vi "XY Plot Commands W2D.vi"(0 "wavenames":string[](array[string])=["'IV0_summ.itx.0003'[0][0]", "'IV0_summ.itx.0003'[0][1]", "'IV0_summ.itx.0003'[0][2]", "'IV0_summ.itx.0003'[0][3]", "'IV0_summ.itx.0003'[0][4]", "'IV0_summ.itx.0003'[0][5]", "'IV0_summ.itx.0003'[0][6]", "'IV0_summ.itx.0003'[0][7]", "'IV0_summ.itx.0003'[0][8]", "'IV0_summ.itx.0003'[0][9]", "'IV0_summ.itx.0003'[0][10]", "'IV0_summ.itx.0003'[0][11]", "'IV0_summ.itx.0003'[0][12]", "'IV0_summ.itx.0003'[0][13]", "'IV0_summ.itx.0003'[0][14]", "'IV0_summ.itx.0003'[0][15]", "'IV0_summ.itx.0003'[0][16]", "'IV0_summ.itx.0003'[0][17]", "'IV0_summ.itx.0003'[0][18]", "'IV0_summ.itx.0003'[0][19]", "'IV0_summ.itx.0003'[0][20]"], 1 "X label":string="energy (eV)", 2 "Y label":string="amplitude (arb)", 3 "input string":string="Display #wave# vs '#waveX#'\nAppendToGraph #wave# vs '#waveX#'\nLabel bottom \"#labelX#\"\nLabel left \"#labelY#\"\nModifyGraph rgb(#wave#)=(#r#,#g#,#b#)\nLegend/C/N=text0\nModifyGraph mirror=1", 4 "X wave":string="x_") -> (5 "result string":string="Display 'IV0_summ.itx.0003'[0][0] vs 'x_'\nAppendToGraph 'IV0_summ.itx.0003'[0][1] vs 'x_'\nAppendToGraph 'IV0_summ.itx.0003'[0][2] vs 'x_'\nAppendToGraph 'IV0_summ.itx.0003'[0][3] vs 'x_'\nAppendToGraph 'IV0_summ.itx.0003'[0][4] vs 'x_'\nAppendToGraph 'IV0_summ.itx.0003'[0][5] vs 'x_'\nAppendToGraph 'IV0_summ.itx.0003'[0][6] vs 'x_'\nAppendToGraph 'IV0_summ.itx.0003'[0][7] vs 'x_'\nAppendToGraph 'IV0_summ.itx.0003'[0][8] vs 'x_'\nAppendToGraph 'IV0_summ.itx.0003'[0][9] vs 'x_'\nAppendToGraph 'IV0_summ.itx.0003'[0][10] vs 'x_'\nAppendToGraph 'IV0_summ.itx.0003'[0][11] vs 'x_'\nAppendToGraph 'IV0_summ.itx.0003'[0][12] vs 'x_'\nAppendToGraph 'IV0_summ.itx.0003'[0][13] vs 'x_'\nAppendToGraph 'IV0_summ.itx.0003'[0][14] vs 'x_'\nAppendToGraph 'IV0_summ.itx.0003'[0][15] vs 'x_'\nAppendToGraph 'IV0_summ.itx.0003'[0][16] vs 'x_'\nAppendToGraph 'IV0_summ.itx.0003'[0][17] vs 'x_'\nAppendToGraph 'IV0_summ.itx.0003'[0][18] vs 'x_'\nAppendToGraph 'IV0_summ.itx.0003'[0][19] vs 'x_'\nAppendToGraph 'IV0_summ.itx.0003'[0][20] vs 'x_'\nLabel bottom \"energy (eV)\"\nLabel left \"amplitude (arb)\"\nModifyGraph rgb('IV0_summ.itx.0003'[0][0])=(65280,0,0)\nModifyGraph rgb('IV0_summ.itx.0003'[0][1])=(65280,16896,0)\nModifyGraph rgb('IV0_summ.itx.0003'[0][2])=(65280,33792,0)\nModifyGraph rgb('IV0_summ.itx.0003'[0][3])=(65280,50688,0)\nModifyGraph rgb('IV0_summ.itx.0003'[0][4])=(63488,65280,0)\nModifyGraph rgb('IV0_summ.itx.0003'[0][5])=(46592,65280,0)\nModifyGraph rgb('IV0_summ.itx.0003'[0][6])=(29696,65280,0)\nModifyGraph rgb('IV0_summ.itx.0003'[0][7])=(12800,65280,0)\nModifyGraph rgb('IV0_summ.itx.0003'[0][8])=(0,65280,4096)\nModifyGraph rgb('IV0_summ.itx.0003'[0][9])=(0,65280,20992)\nModifyGraph rgb('IV0_summ.itx.0003'[0][10])=(0,65280,37888)\nModifyGraph rgb('IV0_summ.itx.0003'[0][11])=(0,65280,53248)\nModifyGraph rgb('IV0_summ.itx.0003'[0][12])=(0,60928,65280)\nModifyGraph rgb('IV0_summ.itx.0003'[0][13])=(0,44032,65280)\nModifyGraph rgb('IV0_summ.itx.0003'[0][14])=(0,27136,65280)\nModifyGraph rgb('IV0_summ.itx.0003'[0][15])=(0,10240,65280)\nModifyGraph rgb('IV0_summ.itx.0003'[0][16])=(6656,0,65280)\nModifyGraph rgb('IV0_summ.itx.0003'[0][17])=(23552,0,65280)\nModifyGraph rgb('IV0_summ.itx.0003'[0][18])=(40448,0,65280)\nModifyGraph rgb('IV0_summ.itx.0003'[0][19])=(57344,0,65280)\nModifyGraph rgb('IV0_summ.itx.0003'[0][20])=(65280,0,56832)\nLegend/C/N=text0")   [LabVIEW 2019, in "LV-Data.ITX.lvclass"]
uses:
  LV-Data.ITX.lvclass
  <userlib>/LevyLab/Graph Utilities/graph_utilities.lvclass
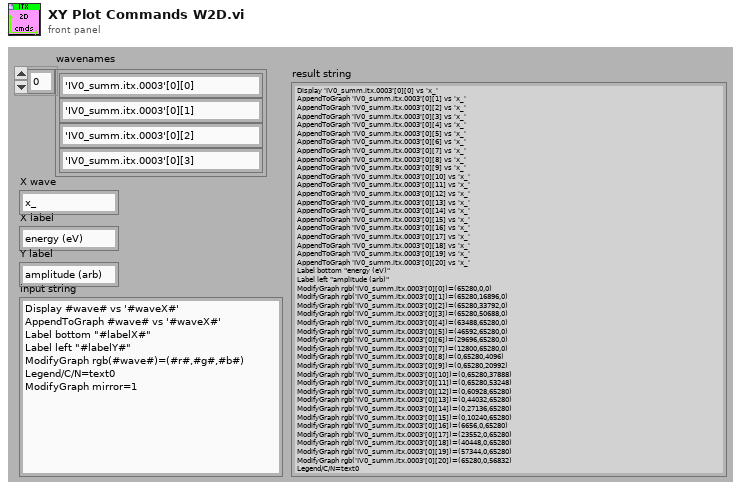
[diagram p1: front panel]
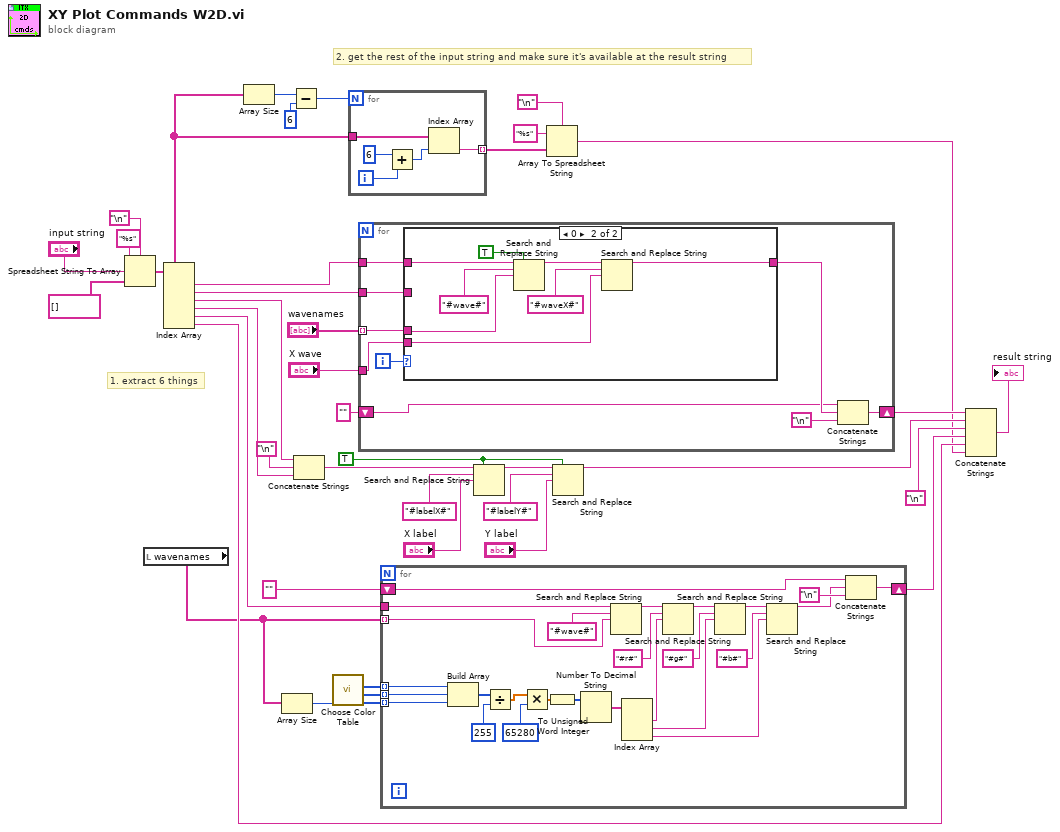
[diagram p0: block diagram]
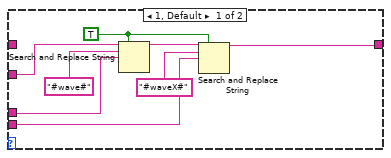
[diagram p2: hidden frame]
diagram:
  w23 = TRUE ("replace all? (F)")
  # "2. get the rest of the input string and make sure it's available at the result string"
  # "1. extract 6 things"
  n1 = Spreadsheet String To Array(delimiter (Tab)="\n", format string="%s", spreadsheet string="input string", array type (2D Dbl)=string[] []) -> (array=w7:string[])
  n2 = local read "wavenames"() -> (w1:string[])
  n3 = Index Array(array=w7) -> (element #1=w31:string, element #2=w30:string, element #3=w14:string, element #4=w15:string, element #5=w16:string, element #6=w17:string)  [unwired: 6 in]
  n4 = Array Size(array=w7) -> (size(s)=w13:i32)
  n5 = Array Size(array=w1) -> (size(s)=w5:i32)
  n6 = Subtract(x=w13, y=6 ("x")) -> (x-y=w11:i32)
  n7 = Concatenate Strings(w14, "\n", w15) -> (w28:string)
  n8 = call <userlib>:"Choose Color Table.vi"("Size (256)"=w5) -> ("B []"=w2:u8[], "G []"=w3:u8[], "R []"=w4:u8[])  [unwired: 7 in, 1 out]
  n9 = for {
    N: w11 -> [_]
    tunnel: w7 -> [w42]
    tunnel: [w41] -> w10 mode=indexing
    i -> [w44]
    n10 = Add(x=6, y=w44) -> (x+y=w45:i32)
    n11 = Index Array(array=w42, index=w45) -> (element=w41:string)
  }
  n12 = for {
    tunnel: "wavenames" -> [w52] mode=indexing
    tunnel: w31 -> [w54]
    tunnel: w30 -> [w53]
    shift-right: [w50] -> w35
    shift-left: "" -> [w47]
    tunnel: "X wave" -> [w46]
    i -> [w51]
    n13 = case shown="0" w51 {
      tunnel: w54 -> [_ w68]
      tunnel: w53 -> [w60 _]
      tunnel: w52 -> [w61 w69]
      tunnel: [w56 w65] -> w49
      tunnel: w46 -> [w57 w63]
      frame 1, Default {
        w55 = TRUE ("replace all? (F)")
        n14 = Search and Replace String(replace all?=w55, input string=w60, search string="#wave#", replace string=w61) -> (result string=w59:string)  [unwired: 1 in, 6 out]
        n15 = Search and Replace String(replace all?=w55, input string=w59, search string="#waveX#", replace string=w57) -> (result string=w56:string)  [unwired: 1 in, 6 out]
      }
      frame 0 {
        n16 = Search and Replace String(replace all?=TRUE ("replace all? (F)"), input string=w68, search string="#wave#", replace string=w69) -> (result string=w66:string)  [unwired: 1 in, 6 out]
        n17 = Search and Replace String(input string=w66, search string="#waveX#", replace string=w63) -> (result string=w65:string)  [unwired: 1 in, 7 out]
      }
    }
    n18 = Concatenate Strings(w47, w49, "\n") -> (w50:string)
  }
  n19 = for {
    tunnel: w16 -> [w89]
    tunnel: w1 -> [w74] mode=indexing
    shift-right: [w85] -> w21
    shift-left: "" -> [w84]
    tunnel: w4 -> [w73] mode=indexing
    tunnel: w3 -> [w72] mode=indexing
    tunnel: w2 -> [w71] mode=indexing
    n20 = Build Array(w73, w72, w71) -> (w96:u8[])
    n21 = Divide(x=w96, y=255) -> (x/y=w92:dbl[])
    n22 = Multiply(x=w92, y=65280) -> (x*y=w93:dbl[])
    n23 = To Unsigned Word Integer(number=w93) -> (unsigned 16bit integer=w91:u16[])
    n24 = Number To Decimal String(number=w91) -> (decimal integer string=w78:string[])  [unwired: 1 out]
    n25 = Search and Replace String(input string=w89, search string="#wave#", replace string=w74) -> (result string=w90:string)  [unwired: 1 in, 7 out]
    n26 = Index Array(array=w78) -> (element #1=w77:string, element #2=w76:string, element #3=w75:string)  [unwired: 3 in]
    n27 = Search and Replace String(input string=w90, search string="#r#", replace string=w77) -> (result string=w88:string)  [unwired: 1 in, 7 out]
    n28 = Search and Replace String(input string=w88, search string="#g#", replace string=w76) -> (result string=w87:string)  [unwired: 1 in, 7 out]
    n29 = Search and Replace String(input string=w87, search string="#b#", replace string=w75) -> (result string=w82:string)  [unwired: 1 in, 7 out]
    n30 = Concatenate Strings(w84, w82, "\n") -> (w85:string)
  }
  n31 = Search and Replace String(replace all?=w23, input string=w28, search string="#labelX#", replace string="X label") -> (result string=w26:string)  [unwired: 1 in, 6 out]
  n32 = Array To Spreadsheet String(delimiter (Tab)="\n", array=w10, 3:"%s" ("format string")) -> (spreadsheet string=w6:string)
  n33 = Search and Replace String(replace all?=w23, input string=w26, search string="#labelY#", replace string="Y label") -> (result string=w19:string)  [unwired: 1 in, 6 out]
  n34 = Concatenate Strings(w35, w19, "\n", w21, w17, w6) -> (→"result string":string)
